vi "FTW-Container-Object-Upsert.vi"(0 "Object in":T1, 5 "Element Name":string, 7 "Container":variant) -> (4 "?":T1, 10 "Found":bool)   [LabVIEW 2015, in "FTW-Container.lvclass"]
uses:
  FTW-Container.lvclass
  FTW-Container-Object.ctl
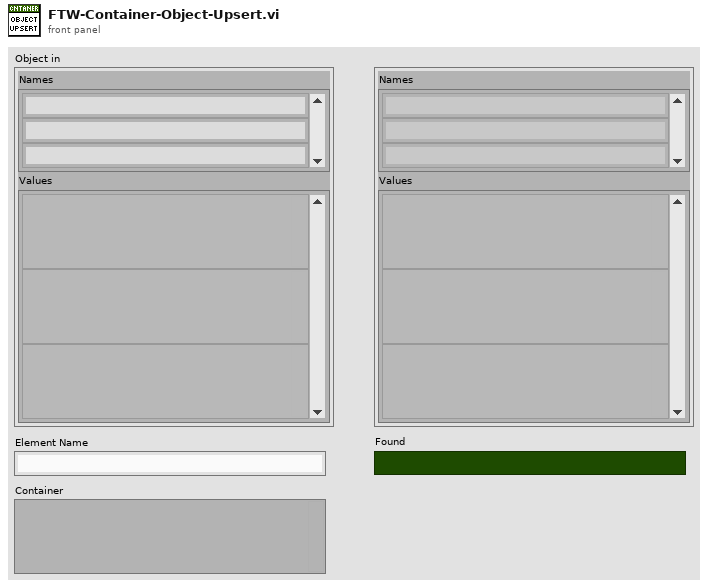
[diagram p1: front panel]
types:
  T1 = typedef "FTW-Container.lvclass/FTW-Container-Object.ctl" = cluster{"Names":string[], "Values":variant[]}
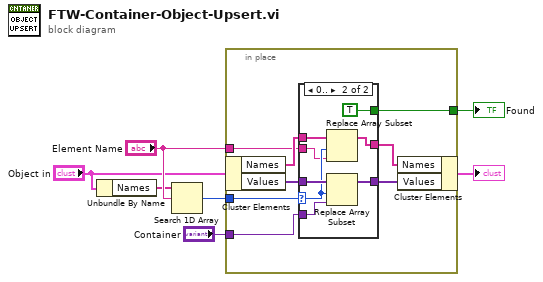
[diagram p0: block diagram]
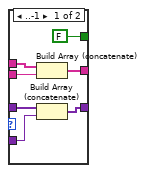
[diagram p2: hidden frame]
diagram:
  n1 = Unbundle By Name("Object in") -> ("Names"=w1:string[])
  n2 = Search 1D Array(1D array=w1, element="Element Name") -> (index of element=w2:i32)  [unwired: 1 in]
  n3 = in-place {
    in-place-border: w2 -> [w11]
    in-place-border: "Element Name" -> [w10]
    in-place-border: "Container" -> [w9]
    in-place-border: [w8] -> w3
    n4 = in-place-cluster #1("Object in") -> ("Names"=w15:string[], "Values"=w13:variant[])
    n5 = case shown="0.." w11 {
      selector: w11 -> [_ w26]
      tunnel: w15 -> [w22 w30]
      tunnel: [w19 w29] -> w14
      tunnel: w13 -> [w21 w28]
      tunnel: [w18 w27] -> w12
      tunnel: w10 -> [w16 w25]
      tunnel: w9 -> [w17 w24]
      tunnel: [FALSE TRUE] -> w8
      frame ..-1 {
        n6 = Build Array (concatenate)(w22, w16) -> (w19:string[])
        n7 = Build Array (concatenate)(w21, w17) -> (w18:variant[])
      }
      frame 0.. {
        n8 = Replace Array Subset(array=w30, new element=w25, index=w26) -> (w29:string[])
        n9 = Replace Array Subset(array=w28, new element=w24, index=w26) -> (w27:variant[])
      }
    }
    n10 = in-place-cluster #1("Names"=w14, "Values"=w12) -> (→"?":T1)
  }
  "Found" <- w3
